vi "Odometry Loop.vi"(6 "error in (no error)":errorcluster) -> ()   [LabVIEW 2019]
uses:
  Typedef/Velocity Data.ctl
  Typedef/Odometry.ctl
  Drive/Pure Pursuit/Typedef/Pure Pursuit Telemetry.ctl
  Drive/Pure Pursuit/Typedef/Path Point.ctl
  <vilib>/Rock Robotics/Network Tables/NT Write Number.vi
  <vilib>/Rock Robotics/Network Tables/NT Write Numeric Array.vi
  Drive/Pure Pursuit/Visualization/Current Path.vi
  Drive/Pure Pursuit/Pure Pursuit.lvlib
panel:
  out "Late Iterations":i16
  out "XY Graph":cluster{dbl[], dbl[]}[](graph)=[{array[1000 elements], array[1000 elements]}, {[-2.247939211922799, 9.450601976465425, 8.114176327244312, -3.5843648611439116, -2.247939211922799], [3.8835413402382706, 1.2106900417960451, -4.638580552398066, -1.9657292539558406, 3.8835413402382706]}, {[0.0, 40.0, 60.0, 100.0], [0.0, 20.0, 80.0, 40.0]}, {array[304 elements], array[304 elements]}, {[7.524752475247524, 1.9801980198019802], [-4.118238955689372, -1.1545613507952672]}, {[-5.727080057823512, -5.705598316147173, -5.641285533198998, -5.534538218672029, -5.386014505257412, -5.196630091037495, -4.967552593902651, -4.700194352798713, -4.396203720187724, -4.057454899406876, -3.686036389581695, -3.28423810933444, -2.8545372786743237, -2.3995831461123918, -1.922180655163488, -1.4252731509367513, -0.9119242334342519, -0.38529886943823066, 0.15135612056157366, 0.6947320800959187, 1.241478915683433, 1.7882257512709472, 2.331601710805292, 2.8682567008050963, 3.3948820648011178, 3.9082309823036177, 4.405138486530354, 4.882540977479257, 5.337495110041189, 5.767195940701306, 6.16899422094856, 6.540412730773742, 6.87916155155459, 7.1831521841655785, 7.450510425269517, 7.679587922404362, 7.86897233662428, 8.017496050038897, 8.124243364565864, 8.18855614751404, 8.210037889190378, 8.18855614751404, 8.124243364565865, 8.017496050038897, 7.86897233662428, 7.679587922404362, 7.450510425269517, 7.18315218416558, 6.879161551554592, 6.540412730773744, 6.168994220948562, 5.76719594070131, 5.337495110041191, 4.882540977479256, 4.405138486530356, 3.9082309823036216, 3.3948820648011195, 2.868256700805095, 2.3316017108052938, 1.788225751270952, 1.2414789156834347, 0.6947320800959172, 0.15135612056157544, -0.3852988694382258, -0.9119242334342501, -1.4252731509367527, -1.9221806551634866, -2.3995831461123878, -2.854537278674323, -3.2842381093344417, -3.686036389581693, -4.057454899406872, -4.396203720187724, -4.700194352798713, -4.967552593902649, -5.196630091037493, -5.386014505257412, -5.534538218672031, -5.641285533198998, -5.705598316147173, -5.727080057823512], [-7.13175642584397, -7.6785032614314845, -8.22187922096583, -8.758534210965633, -9.285159574961655, -9.798508492464155, -10.295415996690892, -10.772818487639794, -11.227772620201726, -11.657473450861843, -12.059271731109098, -12.430690240934279, -12.769439061715127, -13.073429694326116, -13.340787935430054, -13.5698654325649, -13.759249846784815, -13.907773560199434, -14.0145208747264, -14.078833657674576, -14.100315399350915, -14.078833657674576, -14.0145208747264, -13.907773560199434, -13.759249846784817, -13.5698654325649, -13.340787935430054, -13.073429694326116, -12.769439061715127, -12.430690240934279, -12.0592717311091, -11.657473450861843, -11.227772620201728, -10.772818487639796, -10.295415996690892, -9.798508492464155, -9.285159574961655, -8.758534210965635, -8.22187922096583, -7.678503261431485, -7.131756425843971, -6.5850095902564565, -6.041633630722112, -5.504978640722308, -4.978353276726287, -4.465004359223786, -3.9680968549970497, -3.4906943640481467, -3.035740231486214, -2.6060394008260976, -2.2042411205788426, -1.8328226107536638, -1.4940737899728127, -1.1900831573618227, -0.922724916257887, -0.6936474191230433, -0.504263004903124, -0.355739291488506, -0.2489919769615394, -0.18467919401336363, -0.16319745233702498, -0.18467919401336363, -0.24899197696153852, -0.355739291488506, -0.5042630049031231, -0.6936474191230424, -0.9227249162578861, -1.1900831573618218, -1.4940737899728118, -1.832822610753662, -2.2042411205788417, -2.6060394008260923, -3.035740231486211, -3.4906943640481467, -3.9680968549970475, -4.465004359223782, -4.978353276726283, -5.5049786407223085, -6.041633630722109, -6.585009590256451, -7.131756425843968]}]
  out "Drivetrain Chart":T1(graph)
  out "Gyro":dbl(graph)
  out "Encoders":T2(graph)
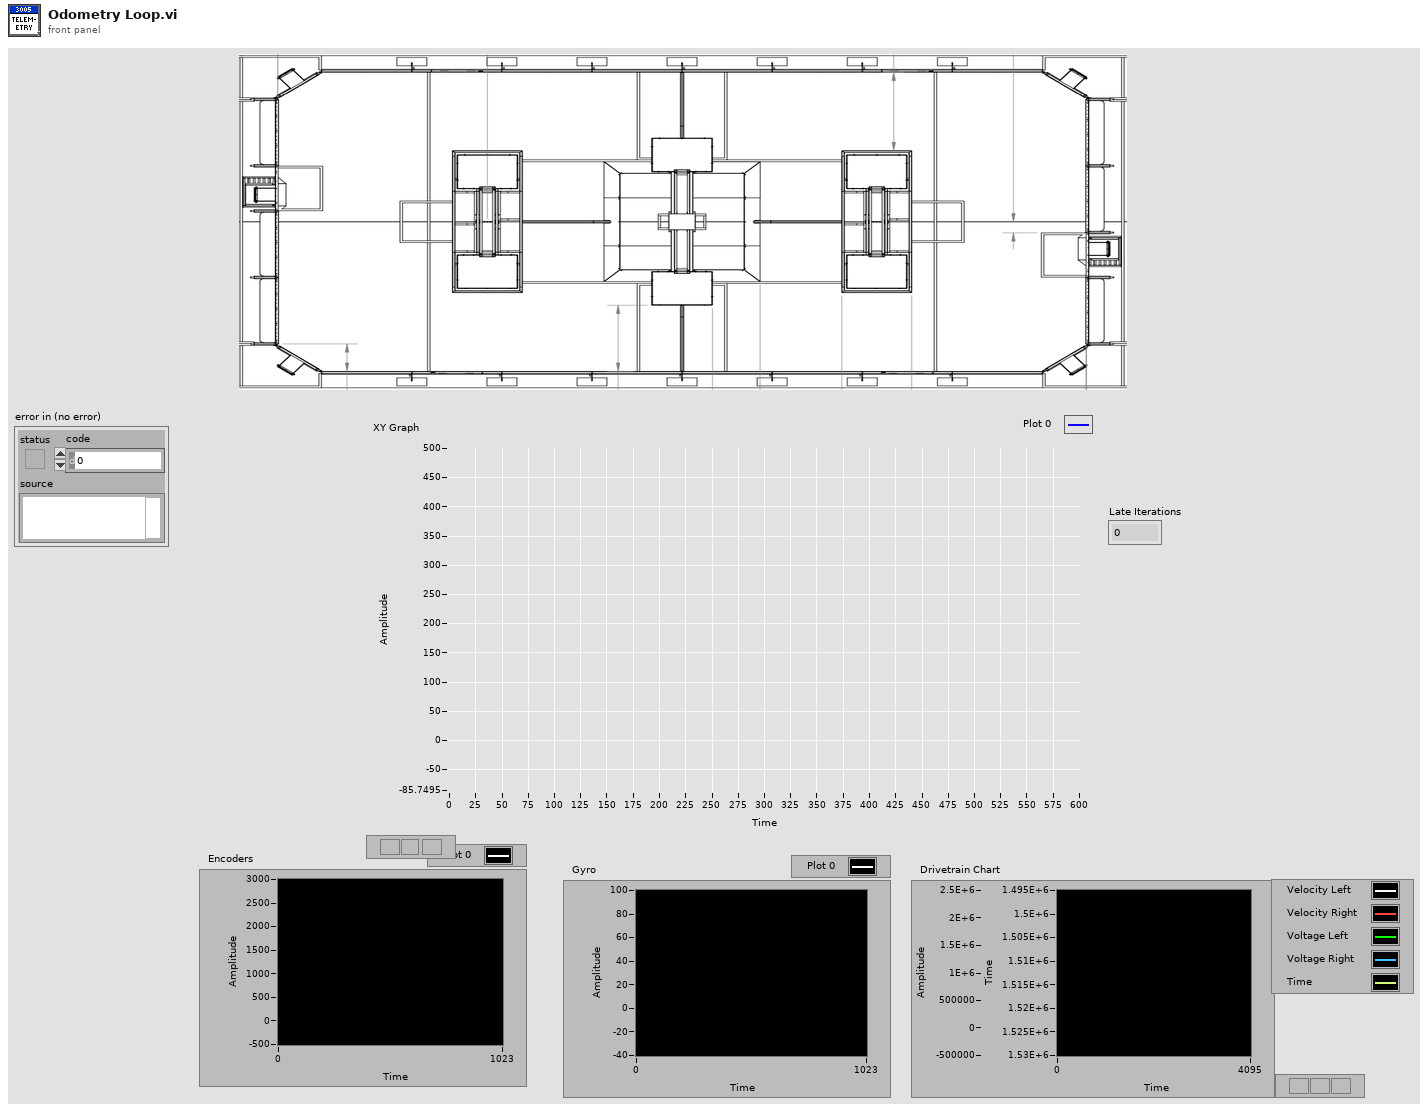
[diagram p1: front panel]
types:
  T1 = cluster{"Left Velocity Raw":sgl, "Right Velocity Raw":sgl, "Voltage":dbl, "Voltage":dbl, "Tick Count(mSec)":u32}
  T2 = cluster{"Left Velocity Raw":sgl, "Right Velocity Raw":sgl}
  T3 = typedef "SPARKMAX6Motor.ctl" = cluster{"FrontLeftMaster":T4, "FrontLeftSlave1":T4, "FrontLeftSlave2":T4, "FrontRightMaster":T4, "FrontRightSlave1":T4, "FrontRightSlave2":T4}
  T4 = typedef "WPI_MotorControlDeviceRef.ctl" = cluster{"DeviceStatus":errorcluster, "Type":T5, "PWM":cluster{"PWM Channel":T6, "DeadBand":T7}, "CAN":cluster{"Device Number":u8, "SetOutput VI Ref":variant, "GetOutput VI Ref":variant, "Enable VI Ref":variant, "Disable VI Ref":variant, "Data":variant}, "Invert":bool, "DIO PWM":cluster{"PWM \"Enable\" Channel":T6, "DIOChannel":T8, "PWM Rate":dbl}}
  T5 = typedef "WPI_MotorControlType.ctl" = enum16{"PWM", "CAN", "DIO PWM"}
  T6 = typedef "FPGA_DIOPWMChannel.ctl" = enum8{"PWM 0", "PWM 1", "PWM 2", "PWM 3", "PWM 4", "PWM 5", "PWM 6", "PWM 7", "PWM 8", "PWM 9", "PWM MXP 0", "PWM MXP 1", "PWM MXP 2", "PWM MXP 3", "PWM MXP 4", "PWM MXP 5", "PWM MXP 6", "PWM MXP 7", "PWM MXP 8", "PWM MXP 9", "Invalid"}
  T7 = typedef "WPI_PWMDeadband.ctl" = cluster{"Name":string, "maxPositivePwm":i32, "minPositivePwm":i32, "centerPwm":i32, "maxNegativePwm":i32, "minNegativePwm":i32, "angularRange":u16}
  T8 = typedef "FPGA_DIOChannel.ctl" = enum8{"DIO 0", "DIO 1", "DIO 2", "DIO 3", "DIO 4", "DIO 5", "DIO 6", "DIO 7", "DIO 8", "DIO 9", "DIO MXP 0", "DIO MXP 1", "DIO MXP 2", "DIO MXP 3", "DIO MXP 4", "DIO MXP 5", "DIO MXP 6", "DIO MXP 7", "DIO MXP 8", "DIO MXP 9", "DIO MXP 10", "DIO MXP 11", "DIO MXP 12", "DIO MXP 13", "DIO MXP 14", "DIO MXP 15", "SPI Port CS1", "SPI Port CS2", "SPI Port CS3", "SPI Port MISO", "SPI Port MOSI", "Invalid"}
  T9 = typedef "Pure Pursuit.lvlib/Pure Pursuit Telemetry.ctl" = cluster{"Target Point":T10, "Close Point":T10, "Curvature":dbl, "index out":i32}
  T10 = typedef "Pure Pursuit.lvlib/Path Point.ctl" = cluster{"x":dbl, "y":dbl, "heading":dbl, "curvature":dbl, "total distance":dbl, "velocity expected":dbl}
  T11 = typedef "Odometry.ctl" = cluster{"x":dbl, "y":dbl, "theta":dbl, "Left Encoder":dbl, "Right Encoder":dbl, "Late Iterations":i16}
  T12 = typedef "Velocity Data.ctl" = cluster{"Right Velocity Raw":sgl, "Left Velocity Raw":sgl}
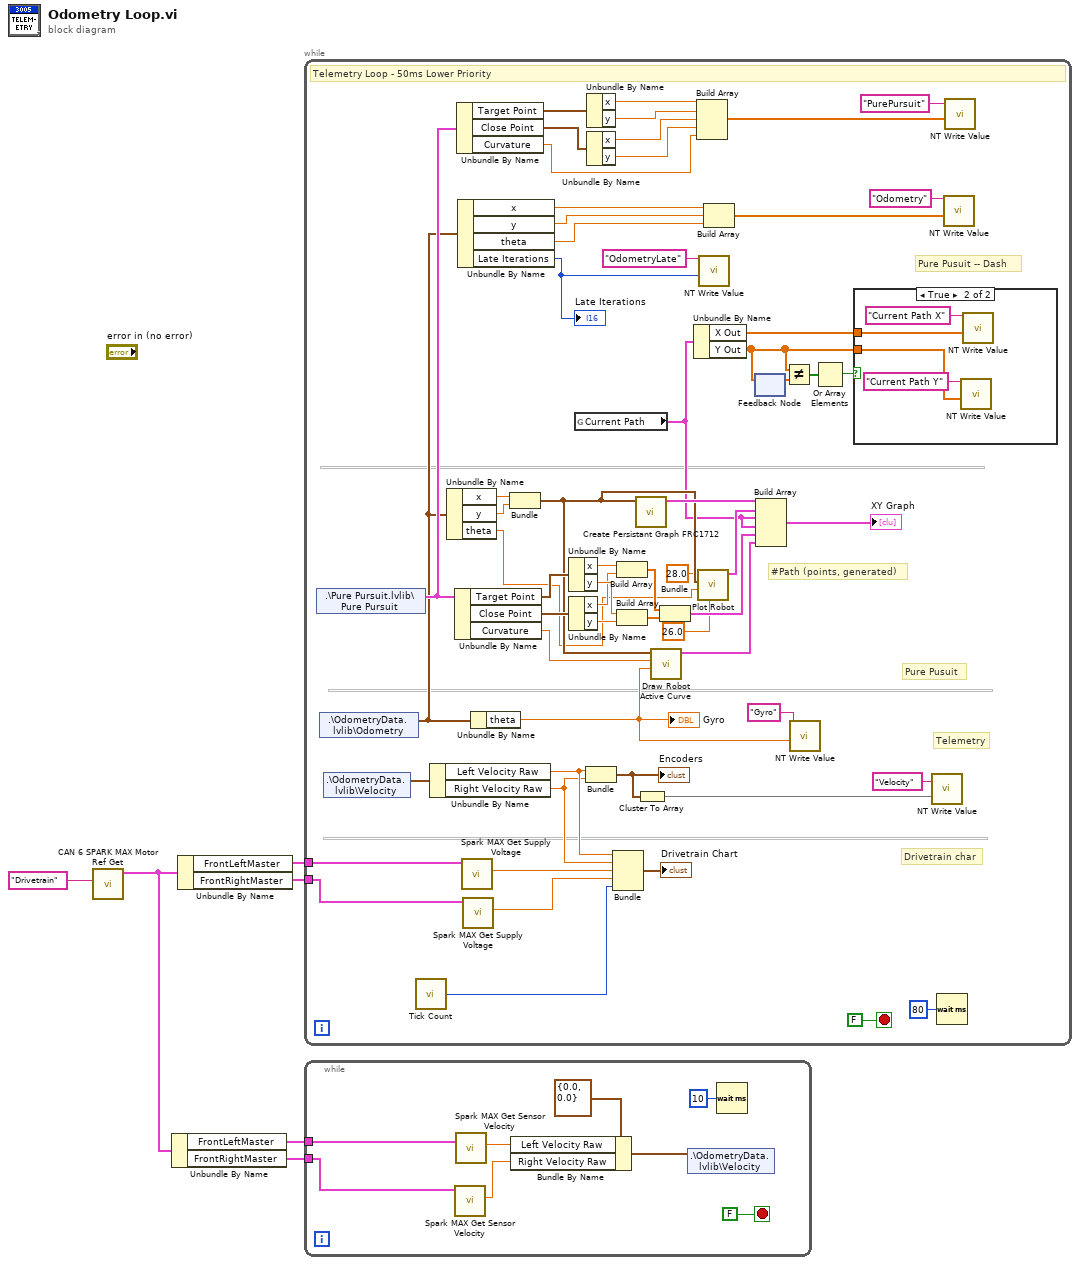
[diagram p0: block diagram]
diagram:
  n1 = call "CAN 6 SPARK MAX Motor Ref Get.vi"("refnum name"="Drivetrain") -> ("TalonSRX6MotorRef out"=w3:T3)  [unwired: 9 in, 1 out]
  n2 = Unbundle By Name(w3) -> ("FrontLeftMaster"=w2:T4, "FrontRightMaster"=w1:T4)
  n3 = Unbundle By Name(w3) -> ("FrontLeftMaster"=w5:T4, "FrontRightMaster"=w4:T4)
  n4 = while {
    tunnel: w5 -> [w13]
    tunnel: w4 -> [w10]
    stop <- FALSE stop-if-true
    # "Pure Pusuit -- Dash"
    # "Telemetry"
    # "Drivetrain char"
    # "Pure Pusuit"
    # "#Path (points, generated)"
    # "Telemetry Loop - 50ms Lower Priority"
    n5 = shared-variable ".\\Pure Pursuit.lvlib\\Pure Pursuit"() -> (w35:T9)  [unwired: 1 in, 1 out]
    n6 = shared-variable ".\\OdometryData.lvlib\\Odometry"() -> (w26:T11)  [unwired: 1 in, 1 out]
    n7 = shared-variable ".\\OdometryData.lvlib\\Velocity"() -> (w9:T12)  [unwired: 1 in, 1 out]
    n8 = call "Tick Count"() -> ("Tick Count(mSec)"=w41:u32)
    n9 = Unbundle By Name(w9) -> ("Left Velocity Raw"=w8:sgl, "Right Velocity Raw"=w7:sgl)
    n10 = Unbundle By Name(w26) -> ("x"=w61:dbl, "y"=w60:dbl, "theta"=w43:dbl)
    n11 = Unbundle By Name(w35) -> ("Target Point"=w50:T10, "Close Point"=w49:T10, "Curvature"=w48:dbl)
    n12 = Unbundle By Name(w35) -> ("Target Point"=w34:T10, "Close Point"=w33:T10, "Curvature"=w28:dbl)
    n13 = Unbundle By Name(w26) -> ("x"=w25:dbl, "y"=w24:dbl, "theta"=w23:dbl, "Late Iterations"=w14:i16)
    "Late Iterations" <- w14
    n14 = call <vilib>:"Spark MAX Get Supply Voltage.vi"("MotorControlDevRef in"=w13) -> ("Voltage"=w12:dbl)  [unwired: 7 in, 3 out]
    n15 = call <vilib>:"Spark MAX Get Supply Voltage.vi"("MotorControlDevRef in"=w10) -> ("Voltage"=w11:dbl)  [unwired: 7 in, 3 out]
    n16 = Unbundle By Name(w26) -> ("theta"=w46:dbl)
    "Gyro" <- w46
    n17 = Bundle("x"=w61, "y"=w60) -> (w45:cluster{"x":dbl, "y":dbl})  [unwired: 1 in]
    n18 = Unbundle By Name(w50) -> ("x"=w57:dbl, "y"=w56:dbl)
    n19 = Unbundle By Name(w49) -> ("x"=w53:dbl, "y"=w52:dbl)
    n20 = global read "Current Path.vi" "Current Path"() -> (w21:cluster{"X Out":dbl[], "Y Out":dbl[]})
    n21 = Bundle("Left Velocity Raw"=w8, "Right Velocity Raw"=w7) -> (w39:T2)  [unwired: 1 in]
    "Encoders" <- w39
    n22 = Unbundle By Name(w34) -> ("x"=w32:dbl, "y"=w31:dbl)
    n23 = Unbundle By Name(w33) -> ("x"=w30:dbl, "y"=w29:dbl)
    n24 = Bundle("Left Velocity Raw"=w8, "Right Velocity Raw"=w7, "Voltage"=w12, "Voltage"=w11, "Tick Count(mSec)"=w41) -> (→"Drivetrain Chart":T1)  [unwired: 1 in]
    n25 = Build Array(w57, w53) -> (w54:dbl[])
    n26 = Build Array(w56, w52) -> (w55:dbl[])
    n27 = call "Create Persistant Graph FRC1712.vi"("XY"=w45) -> ("Graph Plot"=w64:cluster{dbl[], dbl[]})  [unwired: 10 in]
    n28 = Cluster To Array(cluster=w39) -> (array=w38:sgl[])
    n29 = call "Draw Robot Active Curve.vi"("theta"=w46, "Curvature"=w48, "Cluster"=w45) -> ("circle"=w47:cluster{dbl[], dbl[]})  [unwired: 8 in]
    n30 = Bundle(w54, w55) -> (w51:cluster{dbl[], dbl[]})  [unwired: 1 in]
    n31 = Unbundle By Name(w21) -> ("X Out"=w20:dbl[], "Y Out"=w18:dbl[])
    n32 = Build Array(w32, w31, w30, w29, w28) -> (w27:dbl[])
    n33 = call "Plot Robot.vi"("Length"=26.0, "Angle"=w43, "Location"=w45, "Width"=28.0) -> ("Cluster"=w58:cluster{"X Out":dbl[], "Y Out":dbl[]})  [unwired: 7 in]
    n34 = call-poly <vilib>:"NT Write Value.vi"("Numeric"=w14, "Name"="OdometryLate") -> ()  [unwired: 9 in, 1 out]
    n35 = Build Array(w25, w24, w23) -> (w22:dbl[])
    n36 = feedback-in #1(w18) -> ()
    n37 = feedback #1() -> (w19:dbl[])  [unwired: 1 in]
    n38 = Build Array(w64, w58, w21, w21, w51, w47) -> (→"XY Graph":cluster{"X Out":dbl[], "Y Out":dbl[]}[])
    n39 = Not Equal?(x=w18, y=w19) -> (x != y?=w17:bool[])
    n40 = call-poly <vilib>:"NT Write Value.vi"("Numeric"=w46, "Name"="Gyro") -> ()  [unwired: 9 in, 1 out]
    n41 = Or Array Elements(Boolean array=w17) -> (logical OR=w16:bool)
    n42 = case shown="True" w16 {
      tunnel: w18 -> [_ w68]
      tunnel: w20 -> [_ w67]
      frame False {
      }
      frame True {
        n43 = call-poly <vilib>:"NT Write Value.vi"("Numeric Array"=w68, "Name"="Current Path Y") -> ()  [unwired: 9 in, 1 out]
        n44 = call-poly <vilib>:"NT Write Value.vi"("Numeric Array"=w67, "Name"="Current Path X") -> ()  [unwired: 9 in, 1 out]
      }
    }
    n45 = call-poly <vilib>:"NT Write Value.vi"("Numeric Array"=w38, "Name"="Velocity") -> ()  [unwired: 9 in, 1 out]
    n46 = Wait (ms)(milliseconds to wait=u32 80) -> ()  [unwired: 1 out]
    n47 = call-poly <vilib>:"NT Write Value.vi"("Numeric Array"=w22, "Name"="Odometry") -> ()  [unwired: 9 in, 1 out]
    n48 = call-poly <vilib>:"NT Write Value.vi"("Numeric Array"=w27, "Name"="PurePursuit") -> ()  [unwired: 9 in, 1 out]
  }
  n49 = while {
    tunnel: w2 -> [w76]
    tunnel: w1 -> [w75]
    stop <- FALSE stop-if-true
    n50 = call <vilib>:"Spark MAX Get Sensor Velocity.vi"("MotorControlDevRef in"=w75) -> ("Sensor Velocity"=w74:dbl)  [unwired: 7 in, 3 out]
    n51 = call <vilib>:"Spark MAX Get Sensor Velocity.vi"("MotorControlDevRef in"=w76) -> ("Sensor Velocity"=w73:dbl)  [unwired: 7 in, 3 out]
    n52 = Bundle By Name(cluster=T12 {"Right Velocity Raw"=0.0, "Left Velocity Raw"=0.0} ("Velocity"), "Left Velocity Raw"=w73, "Right Velocity Raw"=w74) -> (w72:T12)
    n53 = shared-variable ".\\OdometryData.lvlib\\Velocity"(w72) -> ()  [unwired: 1 in, 1 out]
    n54 = Wait (ms)(milliseconds to wait=u32 10) -> ()  [unwired: 1 out]
  }
